vi "Mutate 1.2.9.vi"(8 "error in (no error)":errorcluster, 11 "Device Ref in":T1 format="%.0x") -> (0 "error out":errorcluster, 3 "Device Ref out":T1 format="%.0x")   [LabVIEW 2019, in "Engine Simulation Toolkit System Explorer.lvlib"]
uses:
  Engine Simulation Toolkit System Explorer.lvlib
  <vilib>/NI VeriStand/Custom Device API/Custom Device Item Ref.ctl
  Shared/Properties.vi
  <vilib>/NI VeriStand/Custom Device API/Get Item Property (Dependent File).vi
  <vilib>/NI VeriStand/Custom Device API/Set Item Property (Dependent File).vi
  Shared/Engine Simulation Toolkit Shared.lvlib
  <vilib>/NI VeriStand/Custom Device API/Custom Device API.lvlib
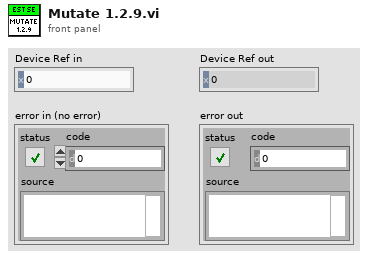
[diagram p1: front panel]
types:
  T1 = typedef "Custom Device API.lvlib/Custom Device Item Ref.ctl" = u64
  T2 = typedef "Custom Device API.lvlib/Dependent File Optional Info.ctl" = cluster{"Version":string, "RTDestination":path, "ForceDownload":bool, "SupportedTarget":string, "MD5":string}
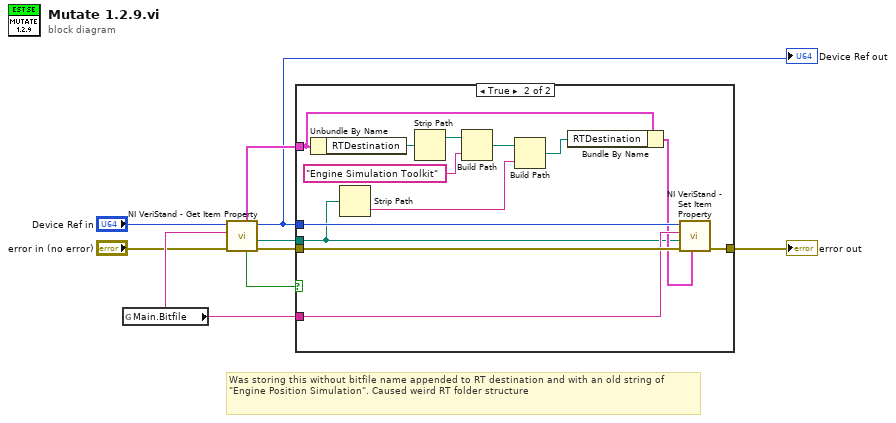
[diagram p0: block diagram]
diagram:
  # "Was storing this without bitfile name appended to RT destination and with an old string of \"Engine Position Simulation\". Caused weird RT folder structure"
  n1 = global read "Properties.vi" "Main.Bitfile"() -> (w5:string)
  n2 = call-poly <vilib>:"NI VeriStand - Get Item Property.vi"("error in (no error)"="error in (no error)", "Property Name"=w5, "Item Ref in"="Device Ref in") -> ("error out"=w4:errorcluster, "Path"=w6:path, "Item Ref out"=w8:T1, "Found"=w3:bool, "OptionalInfo"=w9:T2)  [unwired: 4 in]
  "Device Ref out" <- w8
  n3 = case shown="True" w3 {
    tunnel: w8 -> [_ w23]
    tunnel: w4 -> [w10 w22]
    tunnel: w5 -> [_ w21]
    tunnel: w6 -> [_ w16]
    tunnel: [w10 w20] -> w7
    tunnel: w9 -> [_ w19]
    frame False {
    }
    frame True {
      n4 = Unbundle By Name(w19) -> ("RTDestination"=w15:path)
      n5 = Strip Path(path=w16) -> (name=w17:string)  [unwired: 1 out]
      n6 = Strip Path(path=w15) -> (stripped path=w14:path)  [unwired: 1 out]
      n7 = Build Path(base path=w14, name or relative path="Engine Simulation Toolkit") -> (appended path=w13:path)
      n8 = Build Path(base path=w13, name or relative path=w17) -> (appended path=w11:path)
      n9 = Bundle By Name(cluster=w19, "RTDestination"=w11) -> (w18:T2)
      n10 = call-poly <vilib>:"NI VeriStand - Set Item Property.vi"("OptionalInfo"=w18, "error in (no error)"=w22, "Path"=w16, "Property Name"=w21, "Item Ref in"=w23) -> ("error out"=w20:errorcluster)  [unwired: 4 in, 2 out]
    }
  }
  "error out" <- w7
